vi "DFD Get Cascaded Coef.vi"(7 "type (FLP)":enum16{"FLP", "FXP"}(ring), 8 "error in (no error)":errorcluster, 11 "filter in":T2={"mSRate_Fs"=1.0, "mSRate_Version"="2.0", "mSRate_Comments"="", "mSRate_OrgCoef"={"type"=enum."Undefined", "gain"=1.0, "coef a (k)"=[], "coef b (v)"=[]}, "mSRate_CurCoef"={"type"=enum."Undefined", "gain"=1.0, "coef a (k)"=[], "coef b (v)"=[]}, "mSRate_Quantized?"=FALSE, "mSRate_QCoef"={"type"=enum."Undefined", "gain"=1.0, "coef a (k)"=[], "coef b (v)"=[]}, "mSRate_QSettings"=[], "mSRate_Order"=0, "mSRate_Scaling"={"mSRate_ScaleByPowerOf2?"=FALSE, "mSRate_ScaleType"=enum."No Norm"}} {"mSRate_QSettings"."source" items=["Coef a/k"=0, "Coef b/v"=7, "Input"=1, "Output"=2, "Multiplicand"=3, "Product"=4, "Sum"=5, "Delay"=6, "Gain"=8]}) -> (0 "error out":errorcluster, 1 "gain":dbl, 2 "IIR Filter Cluster":T1, 3 "filter out":T2={"mSRate_Fs"=1.0, "mSRate_Version"="2.0", "mSRate_Comments"="", "mSRate_OrgCoef"={"type"=enum."Undefined", "gain"=1.0, "coef a (k)"=[], "coef b (v)"=[]}, "mSRate_CurCoef"={"type"=enum."Undefined", "gain"=1.0, "coef a (k)"=[], "coef b (v)"=[]}, "mSRate_Quantized?"=FALSE, "mSRate_QCoef"={"type"=enum."Undefined", "gain"=1.0, "coef a (k)"=[], "coef b (v)"=[]}, "mSRate_QSettings"=[], "mSRate_Order"=0, "mSRate_Scaling"={"mSRate_ScaleByPowerOf2?"=FALSE, "mSRate_ScaleType"=enum."No Norm"}} {"mSRate_QSettings"."source" items=["Coef a/k"=0, "Coef b/v"=7, "Input"=1, "Output"=2, "Multiplicand"=3, "Product"=4, "Sum"=5, "Delay"=6, "Gain"=8]})   [LabVIEW 2017, in "NI_DigFilterLicensed.lvlib"]
doc: "Converts a filter to an infinite impulse response (IIR) filter cluster that is compatible with the <B>IIR Filter Cluster</B> output in the Advanced IIR Filtering VIs."
uses:
  <vilib>/addons/Digital Filter Design/NI_DigFilterLicensed.lvlib
  <vilib>/addons/Digital Filter Design/_Objects.llb/DFD Filter Obj.ctl
  <vilib>/addons/Digital Filter Design/_Objects.llb/DFD Filter Coef.ctl
  <vilib>/addons/Digital Filter Design/_Objects.llb/DFD Filter Structure Type Selector.ctl
  <vilib>/addons/Digital Filter Design/_Objects.llb/dfd_Internal Quantization Settings.ctl
  <vilib>/addons/Digital Filter Design/_Objects.llb/dfd_Internal Quantization Srcs.ctl
  <vilib>/addons/Digital Filter Design/_Objects.llb/DFD Coef Norm Type.ctl
  <vilib>/addons/Digital Filter Design/_Objects.llb/DFD Filter Structure Form Id.ctl
  <vilib>/addons/Digital Filter Design/_Misc.llb/dfd_Error Handlers (Single).vi
  <vilib>/addons/Digital Filter Design/FilterLib.llb/dfd_Get Filter Coef Type (Filter IO).vi
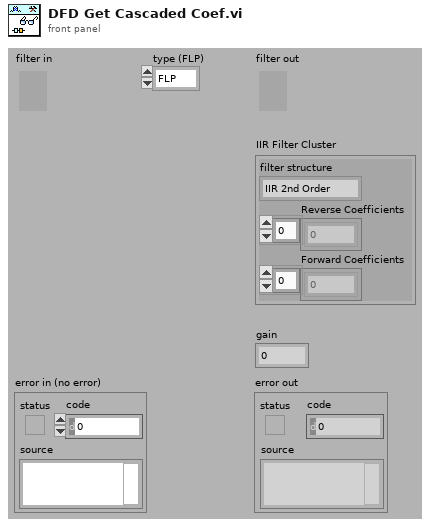
[diagram p1: front panel]
types:
  T1 = cluster{"filter structure":enum32{"IIR 2nd Order", "IIR 4th Order"}, "Reverse Coefficients":dbl[], "Forward Coefficients":dbl[]}
  T2 = typedef "NI_DigFilterLicensed.lvlib/DFD Filter Obj.ctl" = cluster{"mSRate_Fs":dbl, "mSRate_Version":string, "mSRate_Comments":string, "mSRate_OrgCoef":T3, "mSRate_CurCoef":T3, "mSRate_Quantized?":bool, "mSRate_QCoef":T3, "mSRate_QSettings":T5[], "mSRate_Order":i32, "mSRate_Scaling":cluster{"mSRate_ScaleByPowerOf2?":bool, "mSRate_ScaleType":T7}}
  T3 = typedef "NI_DigFilterLicensed.lvlib/DFD Filter Coef.ctl" = cluster{"type":T4, "gain":dbl, "coef a (k)":dbl[], "coef b (v)":dbl[]}
  T4 = typedef "NI_DigFilterLicensed.lvlib/DFD Filter Structure Type Selector.ctl" = enum16{"Undefined", "FIR Direct Form", "FIR Direct Form Transposed", "FIR Symmetric", "FIR Antisymmetric", "IIR Direct Form I", "IIR Direct Form I Transposed", "IIR Direct Form II", "IIR Direct Form II Transposed", "IIR Cascaded Second Order Sections Form I", "IIR Cascaded Second Order Sections Form I Transposed", "IIR Cascaded Second Order Sections Form II", "IIR Cascaded Second Order Sections Form II Transposed", "Lattice Allpass (basic sections)", "Lattice Allpass (one multiplier sections)", "Lattice Allpass (normalized sections)", "Lattice AR (basic sections)", "Lattice AR (one multiplier sections)", "Lattice AR (normalized sections)", "Lattice MA (minimum phase)", "Lattice MA (maximum phase)", "Lattice ARMA (basic sections)", "Lattice ARMA (one multiplier sections)", "Lattice ARMA (normalized sections)"}
  T5 = typedef "NI_DigFilterLicensed.lvlib/dfd_Internal Quantization Settings.ctl" = cluster{"source":T6, "wl":i16, "iwl":i16, "overflow mode":enum16{"Saturation", "Wrap"}, "rounding mode":enum16{"Nearest", "Truncation"}, "signed?":bool}
  T6 = typedef "NI_DigFilterLicensed.lvlib/dfd_Internal Quantization Srcs.ctl" = u16
  T7 = typedef "NI_DigFilterLicensed.lvlib/DFD Coef Norm Type.ctl" = enum16{"No Norm", "Time Domain 1-Norm", "Time Domain 2-Norm", "Time Domain Inf-Norm"}
  T8 = typedef "NI_DigFilterLicensed.lvlib/DFD Filter Structure Form Id.ctl" = enum16{"Undefined", "Direct Form", "SOS Form", "Lattice Form"}
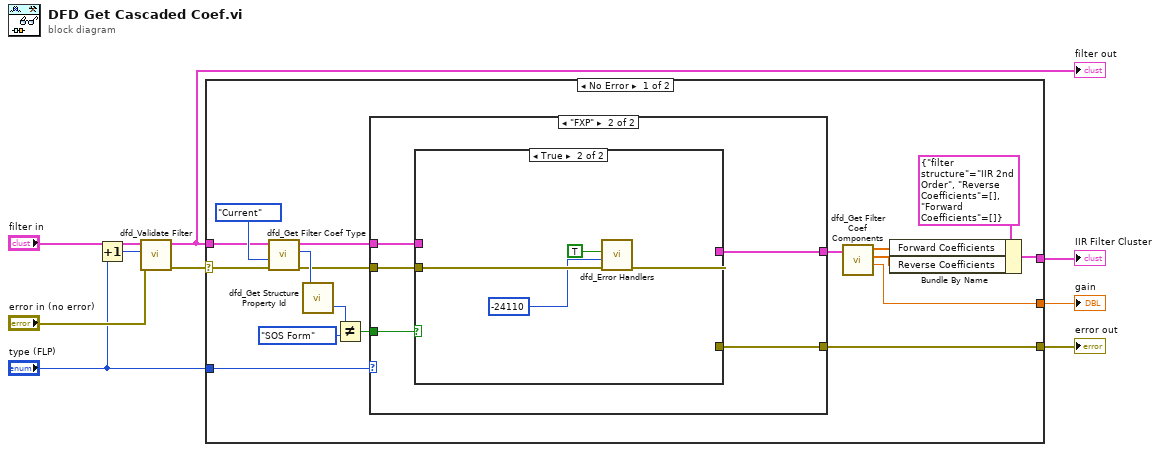
[diagram p0: block diagram]
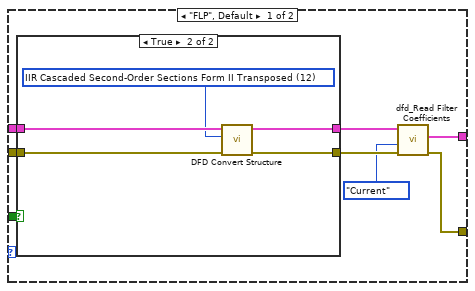
[diagram p2: hidden frame]
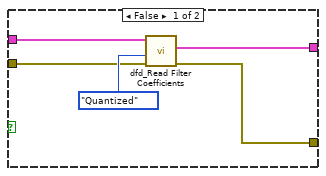
[diagram p4: hidden frame]
diagram:
  n1 = Increment(x="type (FLP)") -> (x+1=w2:enum16{"FLP", "FXP"})
  n2 = call <vilib>:"dfd_Validate Filter.vi"("error in (no error)"="error in (no error)", "check option"=w2, "filter in"="filter in") -> ("error out"=w4:errorcluster, "filter out"=w6:T2)  [unwired: 7 out]
  "filter out" <- w6
  n3 = case shown="No Error" w4 {
    selector: w4 -> [w16 w56]
    tunnel: w6 -> [w17 _]
    tunnel: [w21 w56] -> w9
    tunnel: [w22 _] -> w8
    tunnel: "type (FLP)" -> [w20 _]
    tunnel: [w19 _] -> w3
    frame No Error {
      n4 = call-poly <vilib>:"dfd_Get Filter Coef Type.vi"("error in (no error)"=w16, "coef source"=enum16{"Original", "Current", "Quantized"}."Current", "filter in"=w17) -> ("error out"=w12:errorcluster, "type"=w13:T4, "filter out"=w11:T2)  [unwired: 1 in, 5 out]
      n5 = call <vilib>:"dfd_Get Structure Property Id.vi"("structure type"=w13) -> ("filter structure form id"=w15:T8)  [unwired: 1 out]
      n6 = Not Equal?(x=w15, y=DFD_Filter_Structure_Form_Id."SOS Form" ("filter structure form id")) -> (x != y?=w10:bool)
      n7 = case shown="\"FXP\"" w20 {
        tunnel: w11 -> [w34 w43]
        tunnel: [w33 w44] -> w21
        tunnel: [w32 w42] -> w23
        tunnel: w12 -> [w31 w45]
        tunnel: w10 -> [w27 w46]
        frame "FLP", Default {
          n8 = case shown="True" w27 {
            tunnel: w34 -> [w36 w41]
            tunnel: w31 -> [w35 w40]
            tunnel: [w36 w39] -> w30
            tunnel: [w35 w38] -> w29
            frame False {
            }
            frame True {
              w37 = u16 12 items=["FIR Direct Form"=1, "FIR Direct Form Transposed"=2, "FIR Symmetric"=3, "FIR Antisymmetric"=4, "IIR Direct Form I"=5, "IIR Direct Form I Transposed"=6, "IIR Direct Form II"=7, "IIR Direct Form II Transposed"=8, "IIR Cascaded Second-Order Sections Form I"=9, "IIR Cascaded Second-Order Sections Form I Transposed"=10, "IIR Cascaded Second-Order Sections Form II"=11, "IIR Cascaded Second-Order Sections Form II Transposed"=12, "Lattice Allpass (basic sections)"=13, "Lattice Allpass (one multiplier sections)"=14, "Lattice Allpass (normalized sections)"=15, "Lattice AR (basic sections)"=16, "Lattice AR (one multiplier sections)"=17, "Lattice AR (normalized sections)"=18, "Lattice MA (minimum phase)"=19, "Lattice MA (maximum phase)"=20, "Lattice ARMA (basic sections)"=21, "Lattice ARMA (one multiplier sections)"=22, "Lattice ARMA (normalized sections)"=23] ("target structure")
              n9 = call <vilib>:"DFD Convert Structure.vi"("error in (no error)"=w40, "target structure"=w37, "filter in"=w41) -> ("error out"=w38:errorcluster, "filter out"=w39:T2)  [unwired: 7 out]
            }
          }
          n10 = call <vilib>:"dfd_Read Filter Coefficients.vi"("error in (no error)"=w29, "coef source"=enum16{"Original", "Current", "Quantized"}."Current", "filter in"=w30) -> ("error out"=w33:errorcluster, "filter coef"=w32:T3)  [unwired: 7 out]
        }
        frame "FXP" {
          n11 = case shown="True" w46 {
            tunnel: w45 -> [w49 w55]
            tunnel: [w48 w54] -> w44
            tunnel: w43 -> [w51 _]
            tunnel: [w47 _] -> w42
            frame False {
              n12 = call <vilib>:"dfd_Read Filter Coefficients.vi"("error in (no error)"=w49, "coef source"=enum16{"Original", "Current", "Quantized"}."Quantized", "filter in"=w51) -> ("error out"=w48:errorcluster, "filter coef"=w47:T3)  [unwired: 7 out]
            }
            frame True {
              n13 = call-poly <vilib>:"dfd_Error Handlers.vi"("error in (no error)"=w55, "error code"=-24110 ("ERR_FXP_SOS_EXPECTED"), "condition failed?"=TRUE) -> ("error out"=w54:errorcluster)  [unwired: 8 out]
            }
          }
        }
      }
      n14 = call <vilib>:"dfd_Get Filter Coef Components.vi"("filter coef"=w23) -> ("gain"=w19:dbl, "coef a (k)"=w25:dbl[], "coef b (v)"=w26:dbl[])  [unwired: 1 in, 7 out]
      n15 = Bundle By Name(cluster=T1 {"filter structure"=enum."IIR 2nd Order", "Reverse Coefficients"=[], "Forward Coefficients"=[]} ("IIR Filter Cluster 2"), "Forward Coefficients"=w26, "Reverse Coefficients"=w25) -> (w22:T1)
    }
    frame Error {
    }
  }
  "error out" <- w9
  "IIR Filter Cluster" <- w8
  "gain" <- w3
